vi "Core command.vi"(0 "object in":refnum<class "Serial Device.lvclass">, 1 "Marca":string, 5 "Command":string(combo), 7 "Param 1":string, 9 "Param 2":string, 11 "error in (no error)":errorcluster) -> (4 "object out":refnum<class "Serial Device.lvclass">, 6 "Command":string, 10 "Expected response":string, 15 "error out":errorcluster)   [LabVIEW 2020, in "Serial Device.lvclass"]
uses:
  Serial Device.lvclass
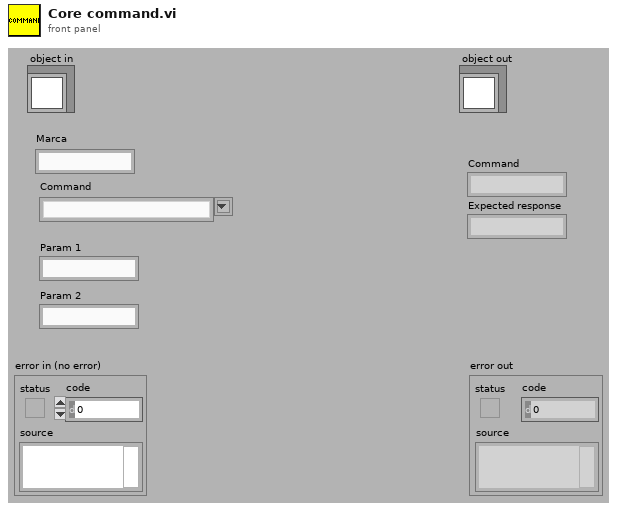
[diagram p1: front panel]
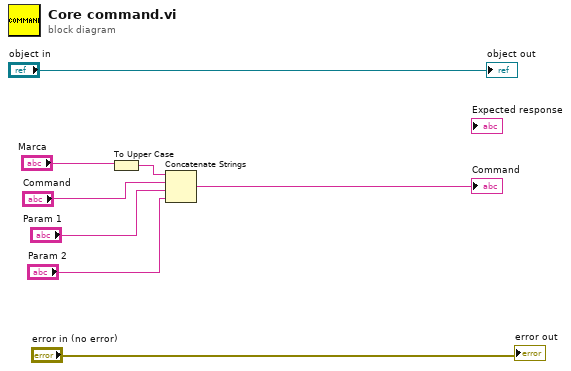
[diagram p0: block diagram]
diagram:
  n1 = To Upper Case(1:"Marca") -> (0:w4:string)
  n2 = Concatenate Strings(w4, "Command", "Param 1", "Param 2") -> (→"Command":string)
  "error out" <- "error in (no error)"
  "object out" <- "object in"
